vi "Shut Down Device.vi"(8 "error in (no error)":errorcluster, 11 "TC-720 in":refnum<class "TC-720.lvclass">) -> (0 "error out":errorcluster, 3 "TC-720 out":refnum<class "TC-720.lvclass">)   [LabVIEW 2023, in "TC-720.lvlib" / "TC-720.lvclass"]
uses:
  TC-720.lvclass
  TC-720.lvclass/TC-720.ctl
  Temperature Controller/Temperature Controller.lvclass
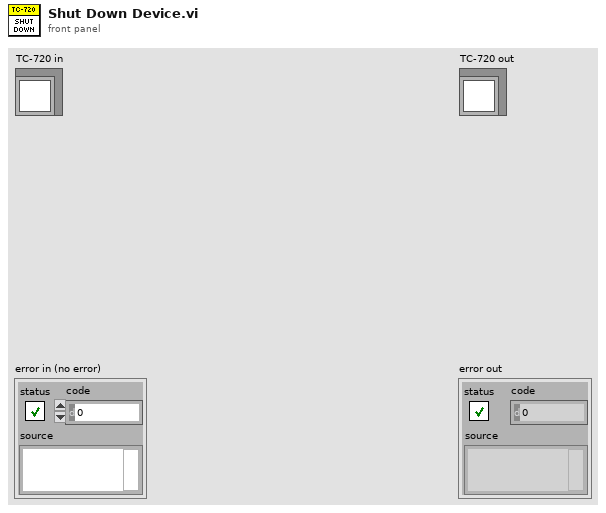
[diagram p1: front panel]
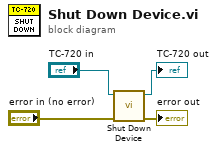
[diagram p0: block diagram]
diagram:
  n1 = call-parent "Shut Down Device.vi"("error in (no error)"="error in (no error)", "Device in"="TC-720 in") -> ("error out"=→"error out":errorcluster, "Device out"=→"TC-720 out":refnum<class "TC-720.lvclass">)  [unwired: 8 in]
